vi "find PUT center.vi"   [LabVIEW 2018]
uses:
  Classes/Workspace/Pick Up Tool Area/Pick Up Tool Fixture.lvclass
  Classes/Controller/Controller.lvclass
  Classes/Routine/Pick and Place/Pick and Place.lvclass
  Classes/Routine/Pick and Place/Pick and Place Type.ctl
types:
  T1 = typedef "Pick and Place.lvclass/Pick and Place Type.ctl" = enum16{"Primary Pick Up", "Secondary Pick Up", "Put Down All", "Pick Up All", "Put Down Secondary"}
  T2 = typedef "Controller.lvclass/Controllers.ctl" = cluster{"I-O.lvclass":refnum<class "I-O.lvclass">, "Gantry":refnum<k24>, "Dispenser":refnum<visa-resource-name>}
  T3 = typedef "Fixture.lvclass/Workspace.ctl" = cluster{"XYZTheta":dbl[], "Workspace Valve":i32, "Workspace Sensor":i32}
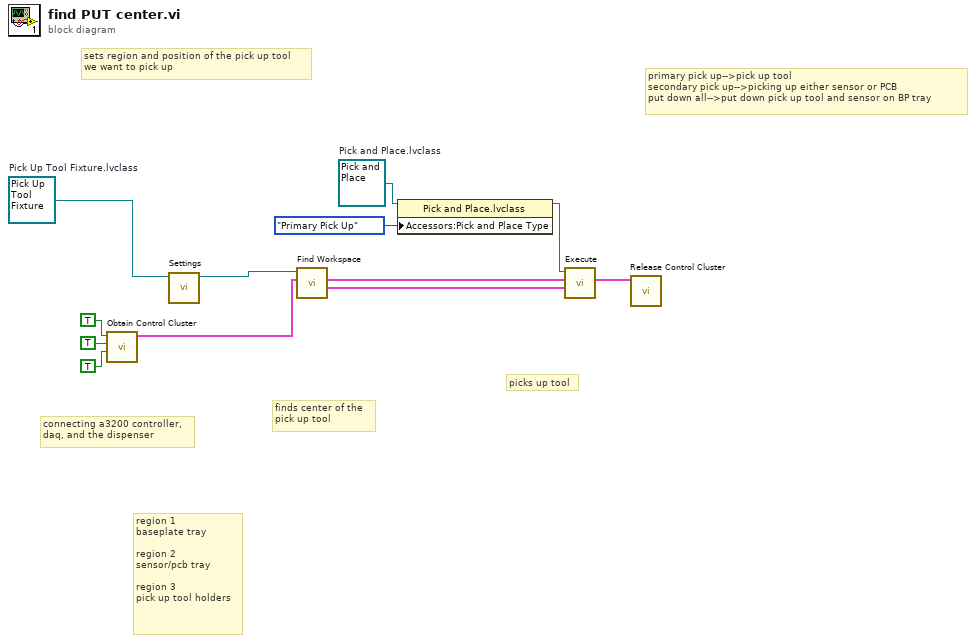
[diagram p0: block diagram]
diagram:
  w9 = refnum<class "Pick and Place.lvclass"> refnum  # Pick and Place.lvclass
  w11 = refnum<class "Pick Up Tool Fixture.lvclass"> refnum  # Pick Up Tool Fixture.lvclass
  # "primary pick up-->pick up tool\nsecondary pick up-->picking up either sensor or PCB\nput down all-->put down pick up tool and sensor on BP tray"
  # "picks up tool"
  # "finds center of the \npick up tool"
  # "connecting a3200 controller,\ndaq, and the dispenser"
  # "region 1\nbaseplate tray\n\nregion 2 \nsensor/pcb tray \n\nregion 3 \npick up tool holders"
  # "sets region and position of the pick up tool\nwe want to pick up"
  n1 = call "Obtain Control Cluster.vi"("I/O"=TRUE, "Dispense"=TRUE, "Motion"=TRUE) -> ("Control Out"=w12:T2)  [unwired: 8 in]
  n2 = call-dynamic "Settings.vi"("Workspace in"=w11) -> ("Workspace out"=w10:refnum<class "Pick Up Tool Fixture.lvclass">)  [unwired: 9 in, 1 out]
  n3 = call-dynamic "Find Workspace.vi"("Control In"=w12, "Workspace In"=w10) -> ("Workspace Out"=w6:T3, "Control Out"=w2:T2)  [unwired: 6 in, 2 out]
  n4 = property class="Pick and Place.lvclass"(reference=w9, "Accessors:Pick and Place Type"=Pick_and_Place_Type."Primary Pick Up" ("Pick and Place Type")) -> (reference out=w7:refnum<class "Pick and Place.lvclass">)  [unwired: 1 in, 1 out]
  n5 = call-dynamic "Execute.vi"("Workspace"=w6, "Cluster"=w2, "Pick and Place in"=w7) -> ("Control Out"=w1:T2)  [unwired: 6 in, 2 out]
  n6 = call "Release Control Cluster.vi"("output cluster"=w1) -> ()  [unwired: 11 in]
